vi "Day10-01_패턴 매칭.vi"(7 "error in":errorcluster) -> (27 "error out":errorcluster)   [LabVIEW 2021]
uses:
  <vilib>/vision/Pattern Matching.llb/IMAQ Curve Parameters.ctl
  <vilib>/vision/Pattern Matching.llb/IMAQ Match Range Setting.ctl
  <vilib>/vision/Pattern Matching.llb/IMAQ Geometric Pattern 2 Advanced Match Options.ctl
panel:
  out "Image":T1(plugin-control)
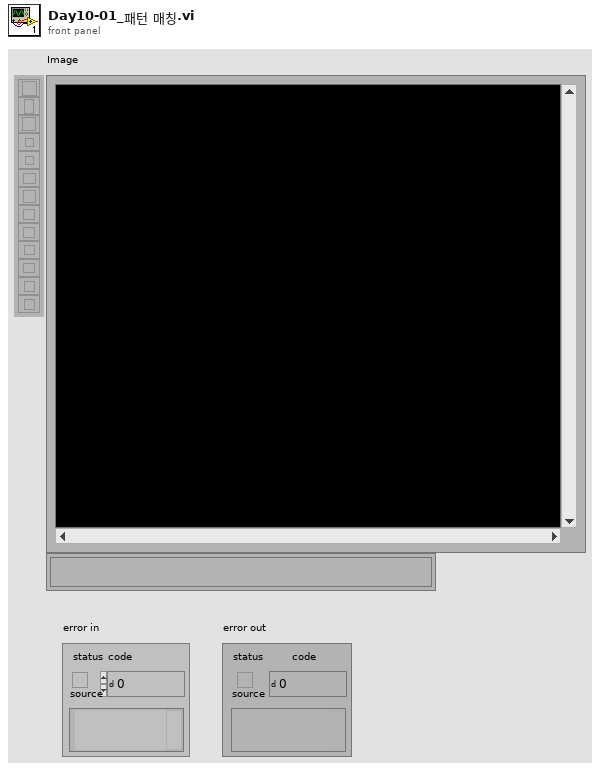
[diagram p1: front panel]
types:
  T1 = typedef "IMAQ Image.ctl" = refnum<image>
  T2 = typedef "IMAQ Curve Parameters.ctl" = cluster{"Extraction Mode":u32, "Edge Threshold":i32, "Edge Filter Size":u32, "Min Length":i32, "Row Search Step Size":i32, "Col Search Step Size":i32, "Max Endpoint Gap":i32, "Closed":bool, "Subpixel":bool}
  T3 = typedef "IMAQ Match Range Setting.ctl" = cluster{"Match Constraints":u32, "Min":dbl, "Max":dbl}
  T4 = typedef "IMAQ Geometric Pattern 2 Advanced Match Options.ctl" = u16
  T5 = cluster{"Curve Parameters":T2, "Match Mode":cluster{"Rotation":bool, "Scale":bool, "Occlusion":bool, "Reserved 1":bool, "Reserved 2":bool, "Reserved 3":bool}, "Range Settings":T3[], "Number of Matches":i32, "Minimum Match Score":sgl, "SubPixel Accuracy":bool, "Adv. Geometric Match Options 2":cluster{"Setup Data Item":T4, "Item Value":dbl}[]}
  T6 = cluster{"Global Rectangle":i32[], "Contours":cluster{"ID":enum32{"External", "Internal"}, "Type":u32, "Coordinates":i32[]}[]}
  T7 = typedef "Image Type" = u32
  T8 = typedef "IMAQ GM Match Report.ctl" = cluster{"Position":cluster{"x":sgl, "y":sgl}, "Angle":sgl, "Scale":sgl, "Score":sgl, "Bounding Box":cluster{"x":sgl, "y":sgl}[], "Contrast Reversed":bool, "Occlusion %":sgl, "Template Target Curve Score":sgl, "Target Template Curve Score":sgl, "Correlation Score":sgl}
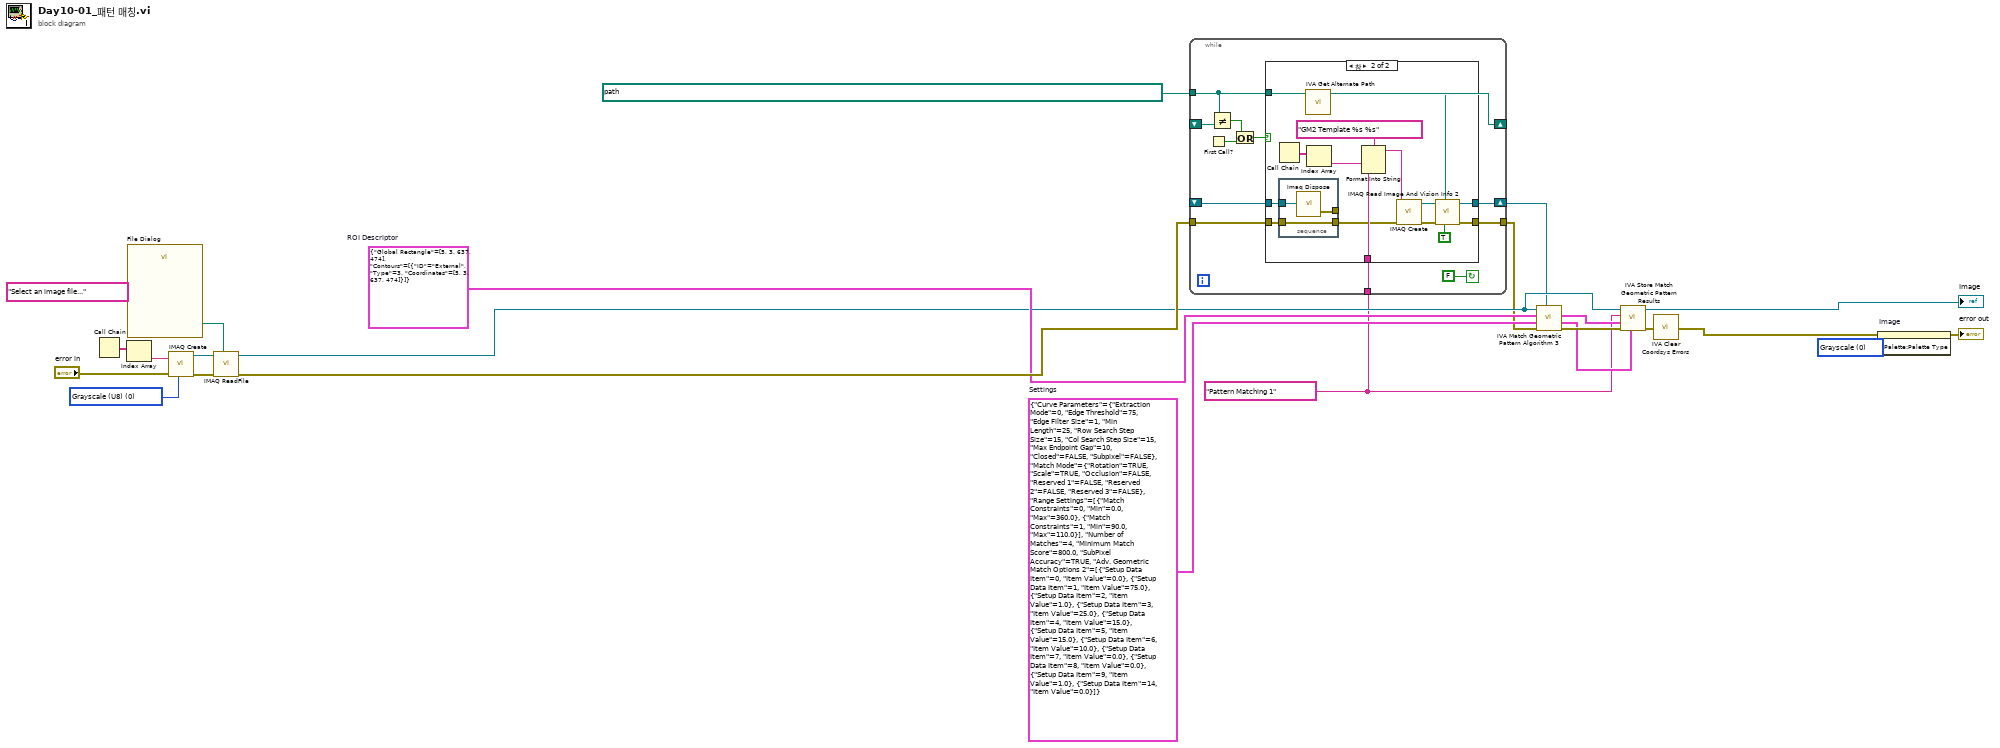
[diagram p0: block diagram]
diagram:
  w1 = u32 0 items=["Grayscale", "Binary", "Gradient", "Rainbow", "Temperature", "User Defined", "Binary 16 Bit", "Gradient 16 Bit", "Rainbow 16 Bit", "Temperature 16 Bit", "User Defined 16 Bit"] ("Palette Type")
  w9 = T5 {"Curve Parameters"={"Extraction Mode"=0, "Edge Threshold"=75, "Edge Filter Size"=1, "Min Length"=25, "Row Search Step Size"=15, "Col Search Step Size"=15, "Max Endpoint Gap"=10, "Closed"=FALSE, "Subpixel"=FALSE}, "Match Mode"={"Rotation"=TRUE, "Scale"=TRUE, "Occlusion"=FALSE, "Reserved 1"=FALSE, "Reserved 2"=FALSE, "Reserved 3"=FALSE}, "Range Settings"=[{"Match Constraints"=0, "Min"=0.0, "Max"=360.0}, {"Match Constraints"=1, "Min"=90.0, "Max"=110.0}], "Number of Matches"=4, "Minimum Match Score"=800.0, "SubPixel Accuracy"=TRUE, "Adv. Geometric Match Options 2"=[{"Setup Data Item"=0, "Item Value"=0.0}, {"Setup Data Item"=1, "Item Value"=75.0}, {"Setup Data Item"=2, "Item Value"=1.0}, {"Setup Data Item"=3, "Item Value"=25.0}, {"Setup Data Item"=4, "Item Value"=15.0}, {"Setup Data Item"=5, "Item Value"=15.0}, {"Setup Data Item"=6, "Item Value"=10.0}, {"Setup Data Item"=7, "Item Value"=0.0}, {"Setup Data Item"=8, "Item Value"=0.0}, {"Setup Data Item"=9, "Item Value"=1.0}, {"Setup Data Item"=14, "Item Value"=0.0}]}  # Settings
  w8 = "Pattern Matching 1" ("Step Name")
  w14 = T6 {"Global Rectangle"=[5, 3, 637, 474], "Contours"=[{"ID"=enum."External", "Type"=3, "Coordinates"=[5, 3, 637, 474]}]}  # ROI Descriptor
  w16 = T7 0 items=["Grayscale (U8)", "Grayscale (I16)", "Grayscale (SGL)", "Complex (CSG)", "RGB (U32)", "HSL (U32)", "RGB (U64)", "Grayscale (U16)"] ("Image Type")
  n1 = Call Chain() -> (call chain=w20:string[])
  n2 = Index Array(array=w20) -> (element=w19:string)  [unwired: 1 in]
  n3 = call "File Dialog"("prompt"="Select an image file...") -> ("selected path"=w17:path)  [unwired: 6 in, 8 out]
  n4 = call "IMAQ Create"("Image Name"=w19, "Image Type"=w16, "error in (no error)"="error in") -> ("New Image"=w23:T1, "error out"=w22:errorcluster)  [unwired: 1 in, 1 out]
  n5 = call "IMAQ ReadFile"("File Path"=w17, "error in (no error)"=w22, "Image"=w23) -> ("error out"=w24:errorcluster, "Image Out"=w10:T1)  [unwired: 2 in, 5 out]
  n6 = while {
    shift-right: [w35] -> w6
    shift-left: _ -> [w34]
    tunnel: [w32] -> w7
    tunnel: w24 -> [w31]
    tunnel: path "C:/Embedded_System/04_LabVIEW/Programming_SourceCode/LabVIEW/Day10_0412/탬플릿2.png" ("Template File Path") -> [w28]
    tunnel: w8 -> [w30]
    shift-right: [w28] -> _
    shift-left: _ -> [w29]
    stop <- FALSE continue-if-true
    n7 = First Call?() -> (First Call?: T/F=w27:bool)
    n8 = Not Equal?(x=w28, y=w29) -> (x != y?=w26:bool)
    n9 = Or(x=w26, y=w27) -> (x .or. y?=w25:bool)
    n10 = case "케이스 구조" shown="참" w25 {
      tunnel: [w37 w39] -> w35
      tunnel: w34 -> [w37 w46]
      tunnel: [w36 w41] -> w32
      tunnel: w31 -> [w36 w47]
      tunnel: w30 -> [_ w48]
      tunnel: w28 -> [_ w45]
      frame False {
      }
      frame True {
        n11 = Call Chain() -> (call chain=w50:string[])
        n12 = stacked-sequence "다층 시퀀스 구조" {
          tunnel: w47 -> [w55]
          tunnel: w46 -> [w54]
          tunnel: [w55] -> w44
          tunnel: [w53] -> _
          frame #0 {
            n13 = call "Imaq Dispose"("Image"=w54) -> ("error out"=w53:errorcluster)  [unwired: 2 in, 3 out]
          }
        }
        n14 = call <vilib>:"IVA Get Alternate Path.vi"("Path In"=w45) -> ("Path Out"=w40:path)  [unwired: 10 out]
        n15 = Index Array(array=w50) -> (element=w49:string)  [unwired: 1 in]
        n16 = Format Into String(format string="GM2 Template %s %s" ("Image Name"), w49, w48) -> (resulting string=w52:string)  [unwired: 2 in, 1 out]
        n17 = call "IMAQ Create"("Image Name"=w52, "error in (no error)"=w44) -> ("New Image"=w38:T1, "error out"=w42:errorcluster)  [unwired: 2 in, 1 out]
        n18 = call "IMAQ Read Image And Vision Info 2"("Use File Path Image Type"=TRUE, "File Path"=w40, "error in (no error)"=w42, "Image"=w38) -> ("error out"=w41:errorcluster, "Image Out"=w39:T1)  [unwired: 5 in, 1 out]
      }
    }
  }
  n19 = call <vilib>:"IVA Match Geometric Pattern Algorithm 3.vi"("Template"=w6, "error in (no error)"=w7, "Settings"=w9, "ROI Descriptor"=w14, "Image"=w10) -> ("error out"=w13:errorcluster, "Calibrated Matches"=w11:T8[], "Matches"=w12:T8[])  [unwired: 4 out]
  n20 = call <vilib>:"IVA Store Match Geometric Pattern Results.vi"("Calibrated Matches"=w11, "error in (no error)"=w13, "Matches"=w12, "Step Name"=w8, "Image in"=w10) -> ("error out"=w5:errorcluster, "Image dup"=→"Image":T1)  [unwired: 5 out]
  n21 = call <vilib>:"IVA Clear Coordsys Errors.vi"("error in (no error)"=w5) -> ("error out"=w4:errorcluster)  [unwired: 10 in]
  n22 = property on="Image" class="ImageControl"(error in=w4, "Palette:Palette Type"=w1) -> (error out=→"error out":errorcluster)  [unwired: 1 in, 1 out]
